vi "PdynToVelocity.vi"() -> ()   [LabVIEW 2014]
doc: "This vi calculates the fluid velocity from the dynamic pressure measured with a pitot tube."
panel:
  out "Air Density (kg/m^3)":dbl format="%#.4g"
  in  "Air Temperature (C)":dbl=20.0
  out "Velocity (fps)":dbl format="%#.1f"
  out "Velocity (m/s)":dbl format="%#.2g"
  in  "Atmospheric Pressure (mBar)":dbl=1000.0
  in  "Pressure Units":string(combo)
  in  "Pdynamic":dbl
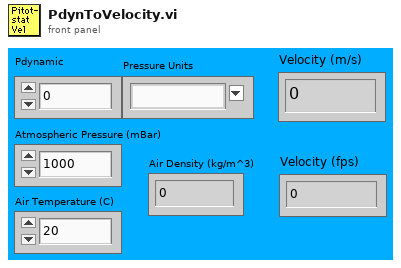
[diagram p1: front panel]
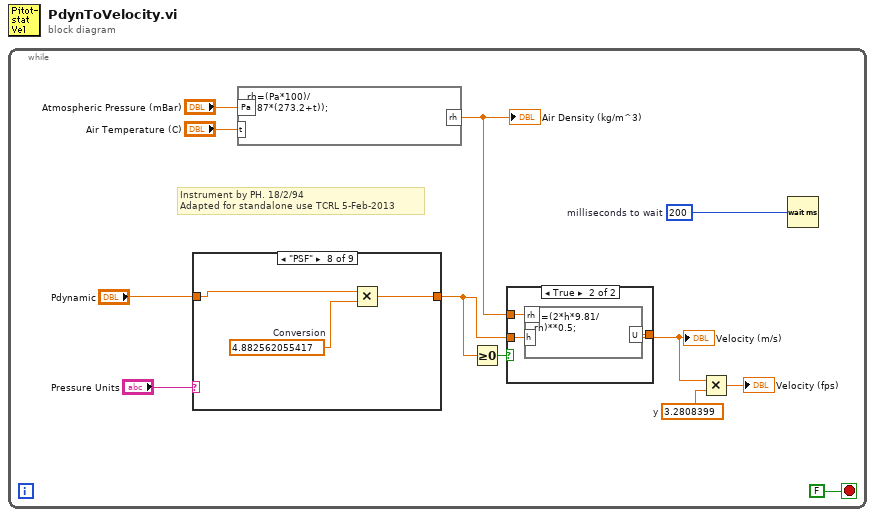
[diagram p0: block diagram]
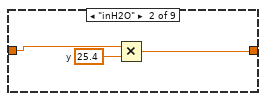
[diagram p3: hidden frame]
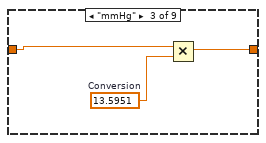
[diagram p4: hidden frame]
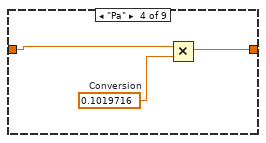
[diagram p5: hidden frame]
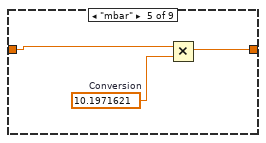
[diagram p6: hidden frame]
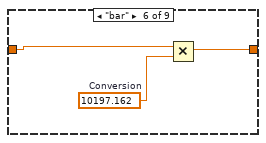
[diagram p7: hidden frame]
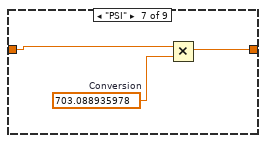
[diagram p8: hidden frame]
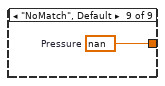
[diagram p9: hidden frame]
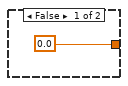
[diagram p10: hidden frame]
diagram:
  n1 = while {
    stop <- FALSE stop-if-true
    w1 = u32 200  # milliseconds to wait
    w5 = 3.2808399  # y
    # "Instrument by PH. 18/2/94\nAdapted for standalone use TCRL 5-Feb-2013"
    n2 = case shown="\"PSF\"" "Pressure Units" {
      tunnel: [w13 w15 w18 w21 w24 w27 w30 w33 w35] -> w11
      tunnel: "Pdynamic" -> [w13 w16 w19 w22 w25 w28 w31 w34 _]
      frame "mmH2O" {
      }
      frame "inH2O" {
        w14 = 25.4  # y
        n3 = Multiply(x=w16, y=w14) -> (x*y=w15:dbl)
      }
      frame "mmHg" {
        w17 = 13.5951  # Conversion
        n4 = Multiply(x=w19, y=w17) -> (x*y=w18:dbl)
      }
      frame "Pa" {
        w20 = 0.1019716  # Conversion
        n5 = Multiply(x=w22, y=w20) -> (x*y=w21:dbl)
      }
      frame "mbar" {
        w23 = 10.1971621  # Conversion
        n6 = Multiply(x=w25, y=w23) -> (x*y=w24:dbl)
      }
      frame "bar" {
        w26 = 10197.162  # Conversion
        n7 = Multiply(x=w28, y=w26) -> (x*y=w27:dbl)
      }
      frame "PSI" {
        w29 = 703.088935978  # Conversion
        n8 = Multiply(x=w31, y=w29) -> (x*y=w30:dbl)
      }
      frame "PSF" {
        w32 = 4.882562055417  # Conversion
        n9 = Multiply(x=w34, y=w32) -> (x*y=w33:dbl)
      }
      frame "NoMatch", Default {
        w35 = nan  # Pressure
      }
    }
    n10 = formula code="rh=(Pa*100)/\n(287*(273.2+t));"("t"="Air Temperature (C)", "Pa"="Atmospheric Pressure (mBar)") -> ("rh"=w3:dbl)
    "Air Density (kg/m^3)" <- w3
    n11 = Greater Or Equal To 0?(x=w11) -> (x >= 0?=w12:bool)
    n12 = case shown="True" w12 {
      tunnel: w3 -> [_ w39]
      tunnel: [0.0 w38] -> w6
      tunnel: w11 -> [_ w37]
      frame False {
      }
      frame True {
        n13 = formula code="U=(2*h*9.81/rh)**0.5;"("rh"=w39, "h"=w37) -> ("U"=w38:dbl)
      }
    }
    "Velocity (m/s)" <- w6
    n14 = Multiply(x=w6, y=w5) -> (x*y=→"Velocity (fps)":dbl)
    n15 = Wait (ms)(milliseconds to wait=w1) -> ()  [unwired: 1 out]
  }
